vi "image ftp.vi"() -> ()   [LabVIEW 2013]
uses:
  <vilib>/FTP/NI_FTP.lvlib
panel:
  out "error out":errorcluster={"status"=FALSE, "code"=221, "source"="221-Goodbye. You uploaded 21 and downloaded 0 kbytes.\r\n221 Logout.\r\n"}
  out "file error":errorcluster
  in  "USER":string="niyantra17@niyantra17-sass.info"
  in  "PASSWORD":string="Sh@shank96"
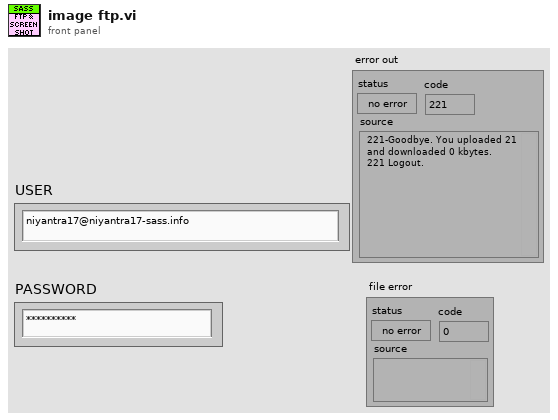
[diagram p1: front panel]
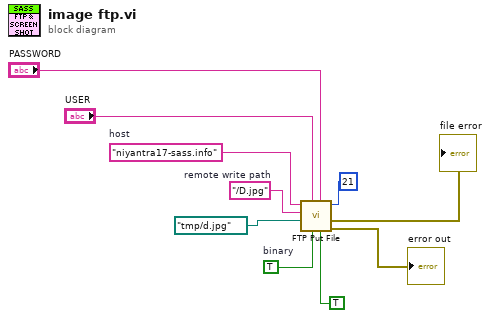
[diagram p0: block diagram]
diagram:
  w8 = TRUE  # binary
  w9 = "/D.jpg"  # remote write path
  w10 = "niyantra17-sass.info"  # host
  n1 = call <vilib>:"FTP Put File.vi"("remote port (21)"=u16 21, "active (T)"=TRUE, "password"="PASSWORD", "binary (F)"=w8, "user"="USER", "local path"=path "/tmp/d.jpg", "remote path"=w9, "host"=w10) -> ("error out"=→"error out":errorcluster, "file error"=→"file error":errorcluster)  [unwired: 2 in]
